vi "Load Section Config Data.vi"(8 "error in (no error)":errorcluster, 9 "delimiter":string=";", 10 "Section":string="Setting", 11 "INI file path":path=path "C:/Workspace/battery-submodule-eol_oop/Config/INI Config.ini") -> (0 "error out":errorcluster, 3 "Data":T1[](array[typedef]))   [LabVIEW 2019, in "Code Modules.lvlib"]
uses:
  Code Modules.lvlib
  Name_values.ctl
  <vilib>/Utility/config.llb/Read Key (String).vi
  <vilib>/Utility/config.llb/NI_LVConfig.lvlib
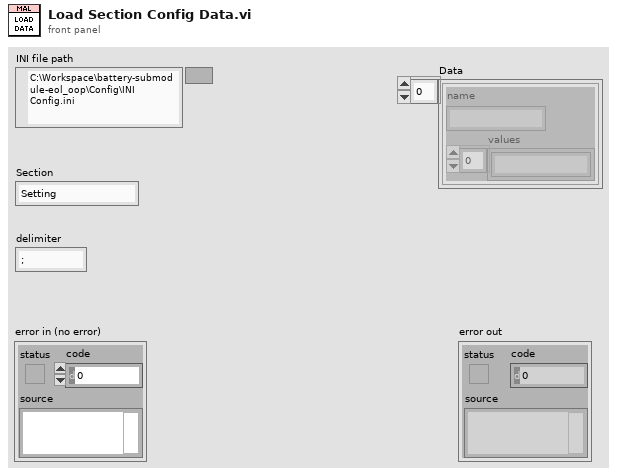
[diagram p1: front panel]
types:
  T1 = typedef "Code Modules.lvlib/Name_values.ctl" = cluster{"name":string, "values":string[]}
  T2 = typedef "NI_LVConfig.lvlib/Config Data RefNum.ctl" = refnum<k1>
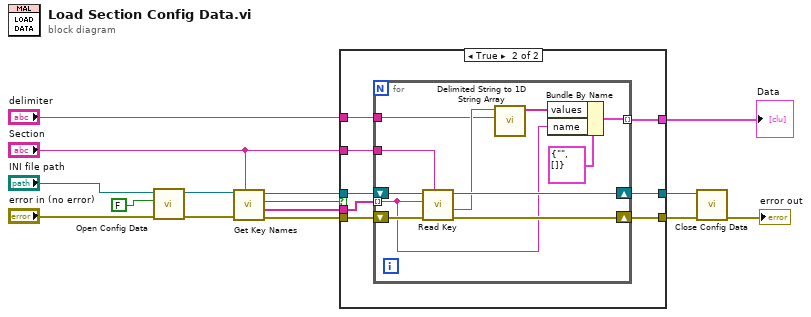
[diagram p0: block diagram]
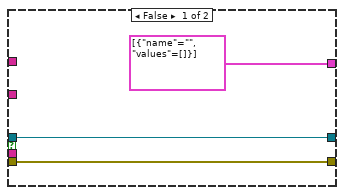
[diagram p2: hidden frame]
diagram:
  n1 = call <vilib>:"Open Config Data.vi"("error in (no error)"="error in (no error)", "create file if necessary (T)"=FALSE, "configuration file path"="INI file path") -> ("error out"=w14:errorcluster, "refnum"=w15:T2)  [unwired: 6 in, 1 out]
  n2 = call <vilib>:"Get Key Names.vi"("section"="Section", "error in (no error)"=w14, "refnum"=w15) -> ("error out"=w12:errorcluster, "key names"=w10:string[], "section exists?"=w13:bool, "refnum out"=w11:T2)  [unwired: 5 in]
  n3 = case shown="True" w13 {
    tunnel: w12 -> [w17 w26]
    tunnel: w11 -> [w18 w25]
    tunnel: w10 -> [_ w24]
    tunnel: "Section" -> [_ w23]
    tunnel: [w17 w22] -> w2
    tunnel: [w18 w21] -> w3
    tunnel: "delimiter" -> [_ w20]
    tunnel: [T1[] [{"name"="", "values"=[]}] w19] -> w1
    frame False {
    }
    frame True {
      n4 = for {
        shift-right: [w35] -> w22
        shift-left: w26 -> [w37]
        tunnel: w24 -> [w29] mode=indexing
        tunnel: w23 -> [w34]
        shift-right: [w33] -> w21
        shift-left: w25 -> [w36]
        tunnel: w20 -> [w31]
        tunnel: [w28] -> w19 mode=indexing
        n5 = call-poly <vilib>:"Read Key.vi"("section"=w34, "error in (no error)"=w37, "key"=w29, "refnum"=w36) -> ("error out"=w35:errorcluster, "value"=w32:string, "refnum out"=w33:T2)  [unwired: 4 in, 1 out]
        n6 = call <vilib>:"Delimited String to 1D String Array.vi"("delimiter"=w31, "delimited string"=w32) -> ("string array"=w30:string[])  [unwired: 9 in]
        n7 = Bundle By Name(cluster=T1 {"name"="", "values"=[]} ("INI Data"), "values"=w30, "name"=w29) -> (w28:T1)
      }
    }
  }
  "Data" <- w1
  n8 = call <vilib>:"Close Config Data.vi"("error in (no error)"=w2, "refnum"=w3) -> ("error out"=→"error out":errorcluster)  [unwired: 8 in, 1 out]
